vi "Read_BSA_data.vi"(0 "GPIB Address":string="13", 7 "No of Check Bytes":i32, 9 "Bytes per block":i32, 11 "error in (no error)":errorcluster) -> (4 "transmission okay":bool, 8 "array of velocity data":u16[](array[numeric]), 15 "error out":errorcluster)   [LabVIEW 2010]
panel:
  out "Loop counter":i32
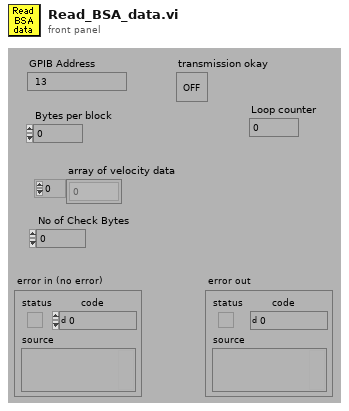
[diagram p1: front panel]
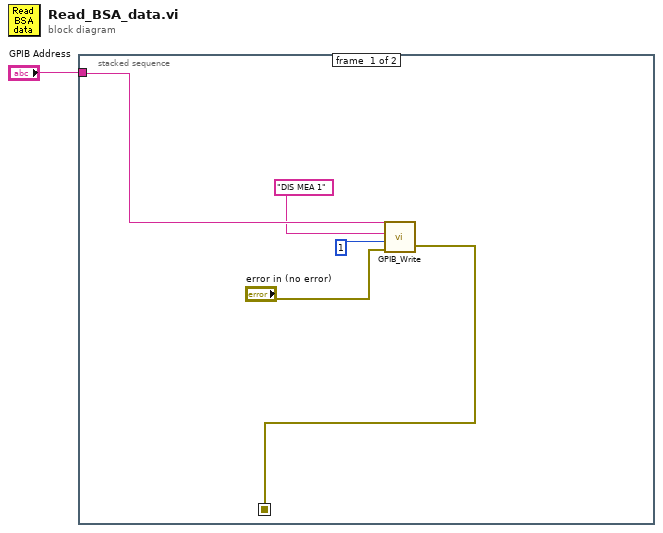
[diagram p0: block diagram]
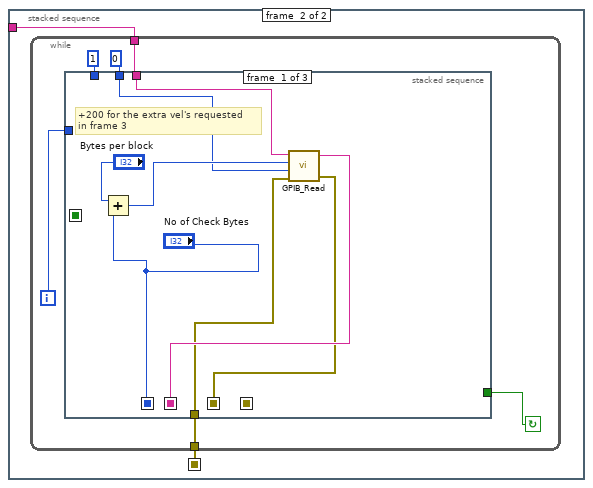
[diagram p2: hidden frame]
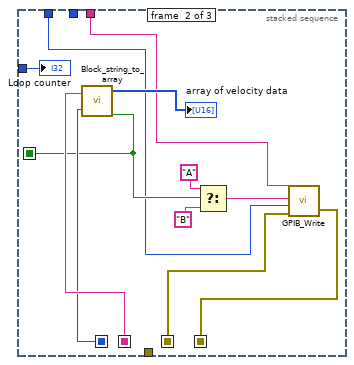
[diagram p3: hidden frame]
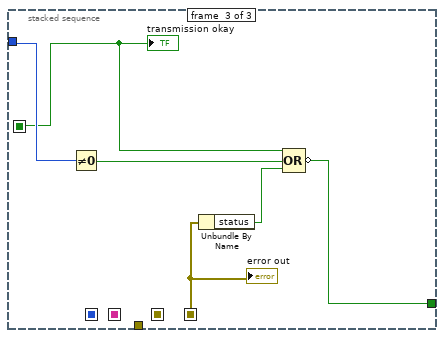
[diagram p4: hidden frame]
diagram:
  n1 = stacked-sequence {
    seq-local: [w2 _] -> [_ w7]
    tunnel: "GPIB Address" -> [w6 w8]
    frame #0 {
      n2 = call "GPIB_Write.vi"("address string"=w6, "data In"="DIS MEA 1", "mode (0)"=i16 1 ("mode"), "error in"="error in (no error)") -> ("error out"=w2:errorcluster)  [unwired: 1 in, 1 out]
    }
    frame #1 {
      n3 = while {
        tunnel: w7 -> [w9]
        tunnel: w8 -> [w14]
        i -> [w11]
        stop <- w10 continue-if-true
        n4 = stacked-sequence {
          seq-local: [w21 _ _] -> [_ w34 _]
          seq-local: ["No of Check Bytes" _ _] -> [_ w33 _]
          seq-local: [_ w30 _] -> [_ _ w39]
          seq-local: [w15 _ _] -> [_ w24 _]
          seq-local: [_ w23 _] -> [_ _ w35]
          tunnel: w14 -> [w22 w26 _]
          tunnel: i16 0 ("Read mode") -> [w19 _ _]
          tunnel: 1 ("Write Mode") -> [_ w25 _]
          tunnel: w11 -> [_ w31 w40]
          tunnel: [_ _ w36] -> w10
          tunnel: w9 -> [w16 _ _]
          frame #0 {
            # "+200 for the extra vel's requested\nin frame 3"
            n5 = Add(x="Bytes per block", y="No of Check Bytes") -> (x+y=w20:i32)
            n6 = call "GPIB_Read.vi"("address string"=w22, "byte count"=w20, "mode (0)"=w19, "error in"=w16) -> ("data Out"=w21:string, "error out"=w15:errorcluster)  [unwired: 1 in, 1 out]
          }
          frame #1 {
            n7 = call "Block_string_to_array.vi"("transmitted string"=w34, "check size"=w33) -> ("array of velocity data"=→"array of velocity data":u16[], "transmission okay"=w30:bool)  [unwired: 1 out]
            n8 = Select(t="A", s=w30, f="B") -> (s? t:f=w27:string)
            n9 = call "GPIB_Write.vi"("address string"=w26, "data In"=w27, "mode (0)"=w25, "error in"=w24) -> ("error out"=w23:errorcluster)  [unwired: 1 in, 1 out]
            "Loop counter" <- w31
          }
          frame #2 {
            n10 = Not Equal To 0?(x=w40) -> (x != 0?=w38:bool)
            n11 = Unbundle By Name(w35) -> ("status"=w37:bool)
            n12 = Compound Arithmetic op=OR(w39, w38, w37) -> (invert w36:bool)
            "transmission okay" <- w39
            "error out" <- w35
          }
        }
      }
    }
  }
